vi "Index uebersetzen.vi"(6 "Aktion":T3, 8 "error in (no error)":errorcluster caption="Fehler (Eingang, kein Fehler)", 9 "Referenz in":sgl, 10 "Index relativ:":u16, 11 "Index Array in":i32[][](array[numeric])) -> (0 "error out":errorcluster caption="Fehler (Ausgang)", 1 "Referenz out":sgl, 2 "Index absolut":i32, 3 "Index Array out":i32[][](array[numeric]), 4 "Komponenten Indices":i32[](array[numeric]), 5 "Komponenten":T1 caption="Cluster")   [LabVIEW 2020, in "EPA 1065.lvlib" / "HovaCAL Interference verificaton.lvlib"]
uses:
  HovaCAL Interference verificaton.lvlib
  Aktion Index uebersetzten.ctl
  Komponenten.ctl
  Visualisierungs Elemente/String - Ausgabefeld.ctl
  Seiten/FT-IR/FGV FT-IR Gasliste Aktionen.ctl
  Aktion FGV Interference.ctl
  Seiten/FT-IR/FT-IR.lvlib
  Linearisierung V2/Gasteiler/Gasteiler.lvlib
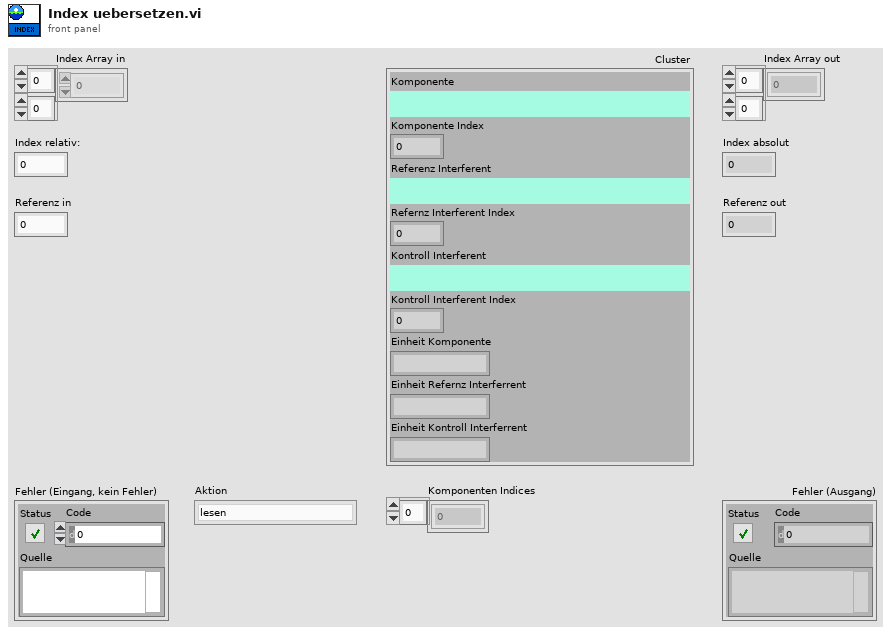
[diagram p1: front panel]
types:
  T1 = typedef "EPA 1065.lvlib/HovaCAL Interference verificaton.lvlib/Komponenten.ctl" = cluster{"Komponente":T2, "Komponente Index":i32, "Referenz Interferent":T2, "Refernz Interferent Index":i32, "Kontroll Interferent":T2, "Kontroll Interferent Index":i32, "Einheit Komponente":string, "Einheit Refernz Interferrent":string, "Einheit Kontroll Interferrent":string}
  T2 = typedef "String - Ausgabefeld.ctl" = string
  T3 = typedef "EPA 1065.lvlib/HovaCAL Interference verificaton.lvlib/Aktion Index uebersetzten.ctl" = enum16{"lesen", "schreiben", "auswerten", "Referenzwert", "KompIndex", "RefInterferIndex", "KontrInterfIndex"}
  T4 = typedef "EPA 1065.lvlib/HovaCAL Interference verificaton.lvlib/Aktion FGV Interference.ctl" = enum16{"Lesen", "TestKonfig", "TestSetting", "Einheiten", "Ergebnis", "Laden", "Tabelle", "Speichern", "löschen"}
  T5 = typedef "FT-IR.lvlib/FGV FT-IR Gasliste Aktionen.ctl" = enum16{"lesen", "Gasliste FT-IR", "Gasliste ausgelesen", "laden", "speichern", "löschen"}
  T6 = typedef "EPA 1065.lvlib/HovaCAL Interference verificaton.lvlib/TestKonfig.ctl" = cluster{"TestKonfig H2O":T7, "TestKonfig Interferent":T13}
  T7 = typedef "EPA 1065.lvlib/HovaCAL Interference verificaton.lvlib/TestKonfig H2O.ctl" = cluster{"Modus":T8, "Komponente:":u16, "Eingangs Konzentration:":dbl, "Einheit":T9, "Anzahl Stufen":sgl, "Zeitdauer Stufen":sgl, "Max Fehler":sgl, "zusätzliche Zeitdauer Erster Punkt":sgl, "Punkte umkehren":bool, "Stufen Tabelle":T10, "HovaCAL Flow Input Cluster":T11, "HovaCAL Temperature":T12}
  T8 = typedef "EPA 1065.lvlib/HovaCAL Interference verificaton.lvlib/Modus.ctl" = u16
  T9 = typedef "Linearisierung v2.lvlib/SpanEinstellungen.lvlib/Einheit.ctl" = enum16{"ppm", "%"}
  T10 = typedef "Linearisierung v2.lvlib/Gasteiler.lvlib/Stufen Tabelle.ctl" = string[][]
  T11 = typedef "Linearisierung v2.lvlib/Gasteiler.lvlib/HovaCAL_Interface.lvlib/Controls.lvlib/Flow Einstellung.ctl" = cluster{"HovaCAL Flow Input Cluster":dbl}
  T12 = typedef "Linearisierung v2.lvlib/Gasteiler.lvlib/HovaCAL_Interface.lvlib/Controls.lvlib/Temp Sollwerte Anzeige.ctl" = dbl[]
  T13 = typedef "EPA 1065.lvlib/HovaCAL Interference verificaton.lvlib/TestKonfig Interferents.ctl" = cluster{"MFC1":enum16{"MFC 1"}, "Eingangs Konzentration MFC1":dbl, "Einheit MFC1 Eingang":T9, "Ausgangs Konzentration MFC1":dbl, "Einheit MFC1 Ausgang":T9, "MFC2":T14, "Referenz-Interferent:":u16, "Gasflaschen Nr MFC2":string, "Eingangs Konzentration MFC2":dbl, "Einheit MFC2 Eingang":T9, "Accuracy MFC2":string, "Ausgangs Konzentration MFC2":dbl, "Einheit MFC2 Ausgang":T9, "MFC3":T14, "Kontroll-Interferent:":u16, "Gasflaschen Nr MFC3":string, "Accuracy MFC3":string, "Eingangs Konzentration MFC3":dbl, "Einheit MFC3 Eingang":T9, "Ausgangs Konzentration MFC3":dbl, "Einheit MFC3 Ausgang":T9, "Gasflasche MFC2":T15, "Gasflasche MFC3":T15}
  T14 = typedef "EPA 1065.lvlib/HovaCAL Interference verificaton.lvlib/MFCAuswahl.ctl" = u16
  T15 = typedef "System Einstellungen V2.lvlib/Gasflasche Auswahl.ctl" = u16
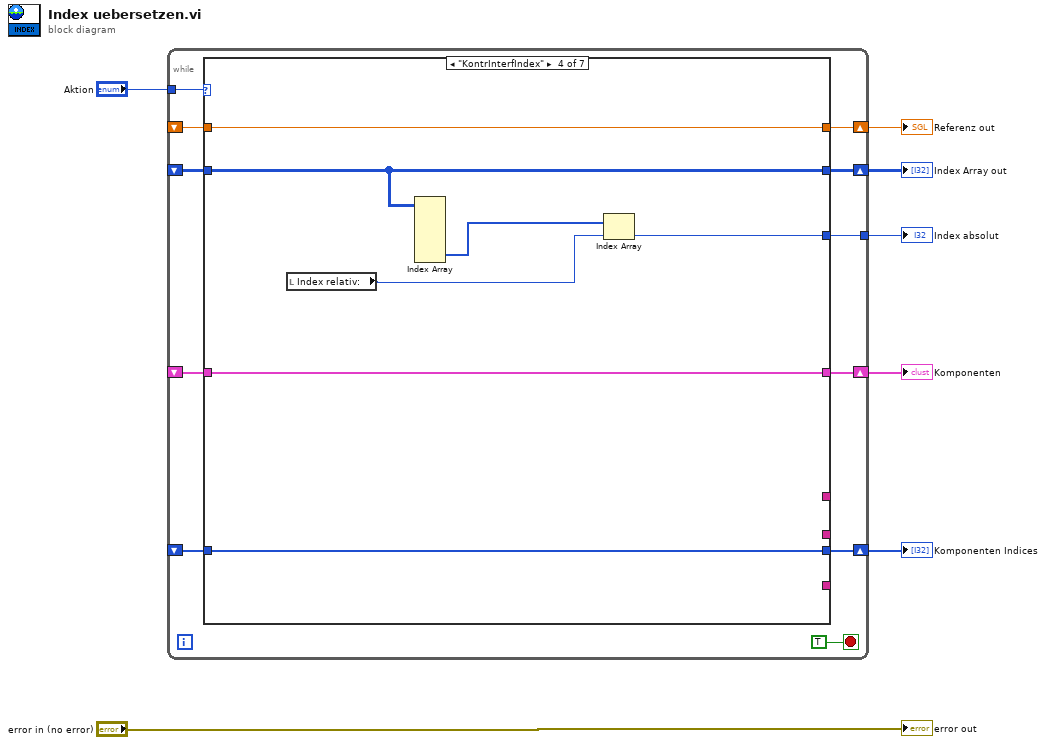
[diagram p0: block diagram]
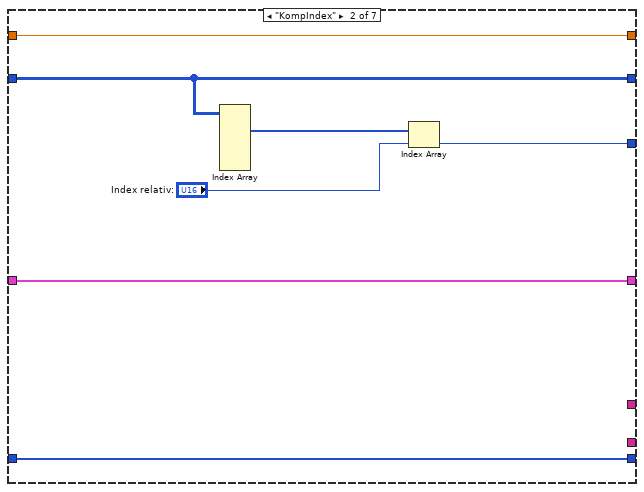
[diagram p3: hidden frame]
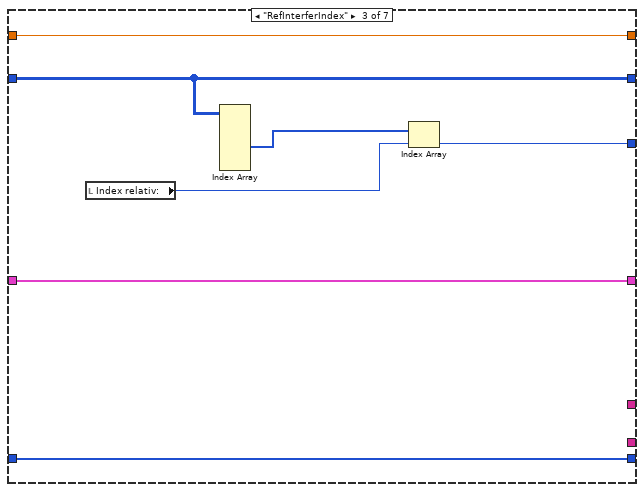
[diagram p4: hidden frame]
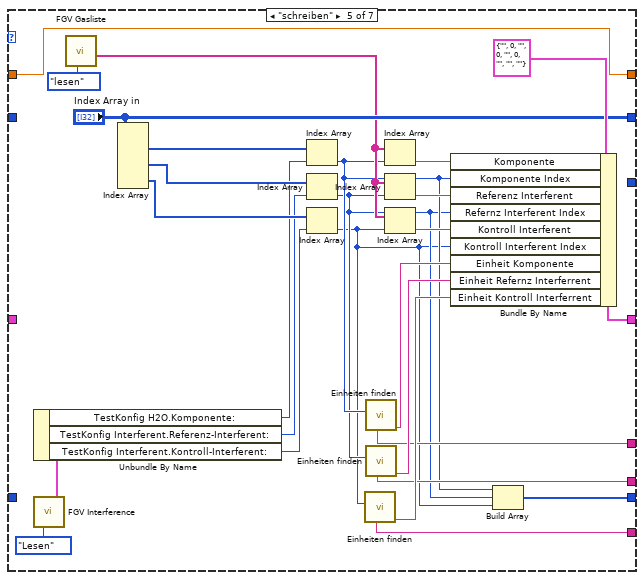
[diagram p5: hidden frame]
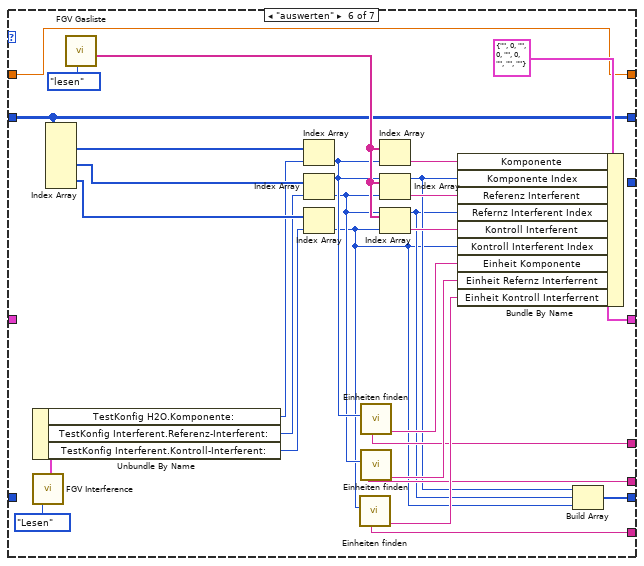
[diagram p6: hidden frame]
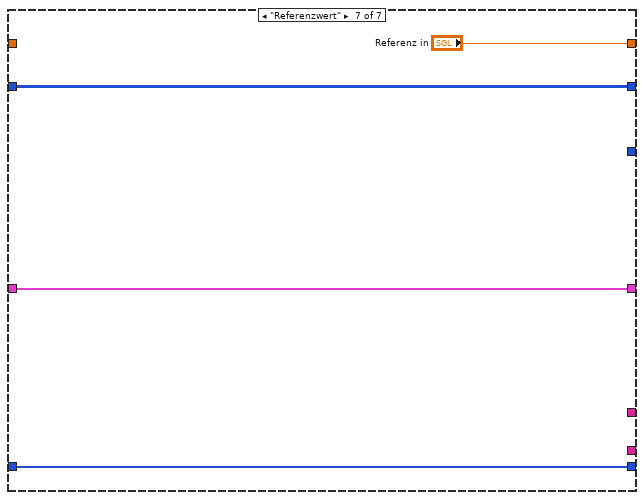
[diagram p7: hidden frame]
diagram:
  n1 = while {
    tunnel: "Aktion" -> [w17]
    shift-right: [w16] -> w6
    shift-left: _ -> [w15]
    shift-right: [w14] -> w2
    shift-left: _ -> [w13]
    shift-right: [w12] -> w5
    shift-left: _ -> [w11]
    shift-right: [w10] -> w3
    shift-left: _ -> [w9]
    tunnel: [w8] -> w1
    stop <- TRUE stop-if-true
    n2 = case shown="\"KontrInterfIndex\"" w17 {
      tunnel: [w22 w29 w36 w43 w66 w93 w99] -> w16
      tunnel: w15 -> [w22 w29 w36 w43 _ _ w99]
      tunnel: [w20 w25 w33 w40 "Index Array in" w86 w100] -> w14
      tunnel: w13 -> [w20 w25 w33 w40 _ w86 w100]
      tunnel: [w21 w28 w35 w42 w60 w88 w98] -> w12
      tunnel: w11 -> [w21 w28 w35 w42 _ _ w98]
      tunnel: [w19 w27 w34 w41 w56 w83 "Referenz in"] -> w10
      tunnel: w9 -> [w19 w27 w34 w41 w56 w83 _]
      tunnel: [_ _ _ _ w49 w76 _] -> _
      tunnel: [_ _ _ _ w48 w75 _] -> _
      tunnel: [_ _ _ _ w47 w74 _] -> _
      tunnel: [_ w23 w32 w39 _ _ _] -> w8
      frame "lesen", Default {
      }
      frame "KompIndex" {
        n3 = Index Array(array=w25) -> (element #1=w26:i32[])  [unwired: 6 in, 2 out]
        n4 = Index Array(array=w26, index="Index relativ:") -> (element=w23:i32)
      }
      frame "RefInterferIndex" {
        n5 = local read "Index relativ:"() -> (w30:u16)
        n6 = Index Array(array=w33) -> (element #2=w31:i32[])  [unwired: 6 in, 2 out]
        n7 = Index Array(array=w31, index=w30) -> (element=w32:i32)
      }
      frame "KontrInterfIndex" {
        n8 = local read "Index relativ:"() -> (w37:u16)
        n9 = Index Array(array=w40) -> (element #3=w38:i32[])  [unwired: 6 in, 2 out]
        n10 = Index Array(array=w38, index=w37) -> (element=w39:i32)
      }
      frame "schreiben" {
        n11 = call "FGV Interference.vi"("Aktion FGV Interference"=Aktion_FGV_Interference."Lesen") -> ("TestKonfig"=w70:T6)  [unwired: 9 in, 5 out]
        n12 = Unbundle By Name(w70) -> ("TestKonfig H2O.Komponente:"=w55:u16, "TestKonfig Interferent.Referenz-Interferent:"=w54:u16, "TestKonfig Interferent.Kontroll-Interferent:"=w53:u16)
        n13 = call "FGV Gasliste.vi"("Aktionen"=FGV_FT-IR_Gasliste_Aktionen."lesen") -> ("Aktuelle Gasliste gesamt"=w59:T2[])  [unwired: 8 in, 2 out]
        n14 = Index Array(array="Index Array in") -> (element #1=w64:i32[], element #2=w62:i32[], element #3=w61:i32[])  [unwired: 6 in]
        n15 = Index Array(array=w64, index=w55) -> (element=w46:i32)
        n16 = Index Array(array=w62, index=w54) -> (element=w45:i32)
        n17 = Index Array(array=w61, index=w53) -> (element=w44:i32)
        n18 = call "Einheiten finden.vi"("Komponente"=w44) -> ("Einheit in String"=w50:string, "Komponenten Name"=w47:T2)  [unwired: 6 in, 3 out]
        n19 = call "Einheiten finden.vi"("Komponente"=w46) -> ("Einheit in String"=w52:string, "Komponenten Name"=w49:T2)  [unwired: 6 in, 3 out]
        n20 = call "Einheiten finden.vi"("Komponente"=w45) -> ("Einheit in String"=w51:string, "Komponenten Name"=w48:T2)  [unwired: 6 in, 3 out]
        n21 = Index Array(array=w59, index=w46) -> (element=w63:T2)
        n22 = Index Array(array=w59, index=w45) -> (element=w58:T2)
        n23 = Index Array(array=w59, index=w44) -> (element=w57:T2)
        n24 = Bundle By Name(cluster=T1 {"Komponente"="", "Komponente Index"=0, "Referenz Interferent"="", "Refernz Interferent Index"=0, "Kontroll Interferent"="", "Kontroll Interferent Index"=0, "Einheit Komponente"="", "Einheit Refernz Interferrent"="", "Einheit Kontroll Interferrent"=""} ("Komponenten"), "Komponente"=w63, "Komponente Index"=w46, "Referenz Interferent"=w58, "Refernz Interferent Index"=w45, "Kontroll Interferent"=w57, "Kontroll Interferent Index"=w44, "Einheit Komponente"=w52, "Einheit Refernz Interferrent"=w51, "Einheit Kontroll Interferrent"=w50) -> (w66:T1)
        n25 = Build Array(w46, w45, w44) -> (w60:i32[])
      }
      frame "auswerten" {
        n26 = call "FGV Interference.vi"("Aktion FGV Interference"=Aktion_FGV_Interference."Lesen") -> ("TestKonfig"=w97:T6)  [unwired: 9 in, 5 out]
        n27 = Unbundle By Name(w97) -> ("TestKonfig H2O.Komponente:"=w82:u16, "TestKonfig Interferent.Referenz-Interferent:"=w81:u16, "TestKonfig Interferent.Kontroll-Interferent:"=w80:u16)
        n28 = Index Array(array=w86) -> (element #1=w92:i32[], element #2=w90:i32[], element #3=w89:i32[])  [unwired: 6 in]
        n29 = call "FGV Gasliste.vi"("Aktionen"=FGV_FT-IR_Gasliste_Aktionen."lesen") -> ("Aktuelle Gasliste gesamt"=w87:T2[])  [unwired: 8 in, 2 out]
        n30 = Index Array(array=w92, index=w82) -> (element=w73:i32)
        n31 = Index Array(array=w90, index=w81) -> (element=w72:i32)
        n32 = Index Array(array=w89, index=w80) -> (element=w71:i32)
        n33 = call "Einheiten finden.vi"("Komponente"=w71) -> ("Einheit in String"=w77:string, "Komponenten Name"=w74:T2)  [unwired: 6 in, 3 out]
        n34 = call "Einheiten finden.vi"("Komponente"=w73) -> ("Einheit in String"=w79:string, "Komponenten Name"=w76:T2)  [unwired: 6 in, 3 out]
        n35 = call "Einheiten finden.vi"("Komponente"=w72) -> ("Einheit in String"=w78:string, "Komponenten Name"=w75:T2)  [unwired: 6 in, 3 out]
        n36 = Index Array(array=w87, index=w73) -> (element=w91:T2)
        n37 = Index Array(array=w87, index=w72) -> (element=w85:T2)
        n38 = Index Array(array=w87, index=w71) -> (element=w84:T2)
        n39 = Bundle By Name(cluster=T1 {"Komponente"="", "Komponente Index"=0, "Referenz Interferent"="", "Refernz Interferent Index"=0, "Kontroll Interferent"="", "Kontroll Interferent Index"=0, "Einheit Komponente"="", "Einheit Refernz Interferrent"="", "Einheit Kontroll Interferrent"=""} ("Komponenten"), "Komponente"=w91, "Komponente Index"=w73, "Referenz Interferent"=w85, "Refernz Interferent Index"=w72, "Kontroll Interferent"=w84, "Kontroll Interferent Index"=w71, "Einheit Komponente"=w79, "Einheit Refernz Interferrent"=w78, "Einheit Kontroll Interferrent"=w77) -> (w93:T1)
        n40 = Build Array(w73, w72, w71) -> (w88:i32[])
      }
      frame "Referenzwert" {
      }
    }
  }
  "Komponenten" <- w6
  "Komponenten Indices" <- w5
  "Referenz out" <- w3
  "Index Array out" <- w2
  "Index absolut" <- w1
  "error out" <- "error in (no error)"
